vi "Console Example.vi"() -> ()   [LabVIEW 2020, in "ase.console.lvlib"]
uses:
  ase.console.lvlib
  <vilib>/Utility/miscctls.llb/LVPointTypeDef.ctl
  ase/ase/ase.lvclass/ase.ctl
  ase/ase/Merge Call Library Errors.vi
  ase/ase/Trim Whitespace.vi
  ase/ase/Check Shared Library Version.vi
  ase/ase/Write Data to Std In.vi
  ase/ase/Error Invalid ASE Handle.vi
  ase/ase/Error Internal Library Implementation Error.vi
  <vilib>/Utility/error.llb/Error Cluster From Error Code.vi
  ase/ase/Wait on Call.vi
  ase/ase/ase.lvclass
panel:
  in  "Write Exit":bool
  in  "Clear Std Out":bool
  in  "Start Console":bool
  in  "Send Terminate":bool
  in  "Clear Std Err":bool
  in  "working directory":path=path "c:/"
  in  "Send":bool
  in  "Cmd":string="echo hello!" caption="Cmd In (can include multiple lines)"
  out "Std Err":string
  out "Std Out":string
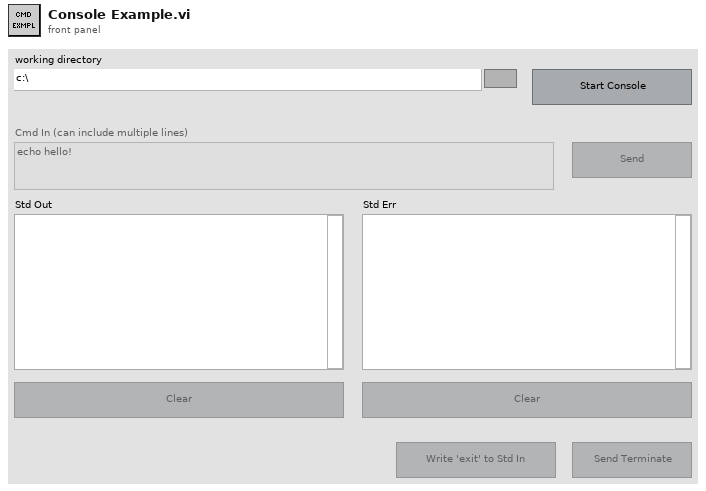
[diagram p1: front panel]
types:
  T1 = enum8{"Enabled", "Disabled", "Disabled and Grayed Out"}
  T2 = typedef "LVPointTypeDef.ctl" = cluster{"Horizontal":i16, "Vertical":i16}
  T3 = typedef "ase.lvlib/ase.lvclass/Event References.ctl" = cluster{"Standard Output":refnum<user-event>, "Standard Error":refnum<user-event>, "Did Exit":refnum<user-event>}
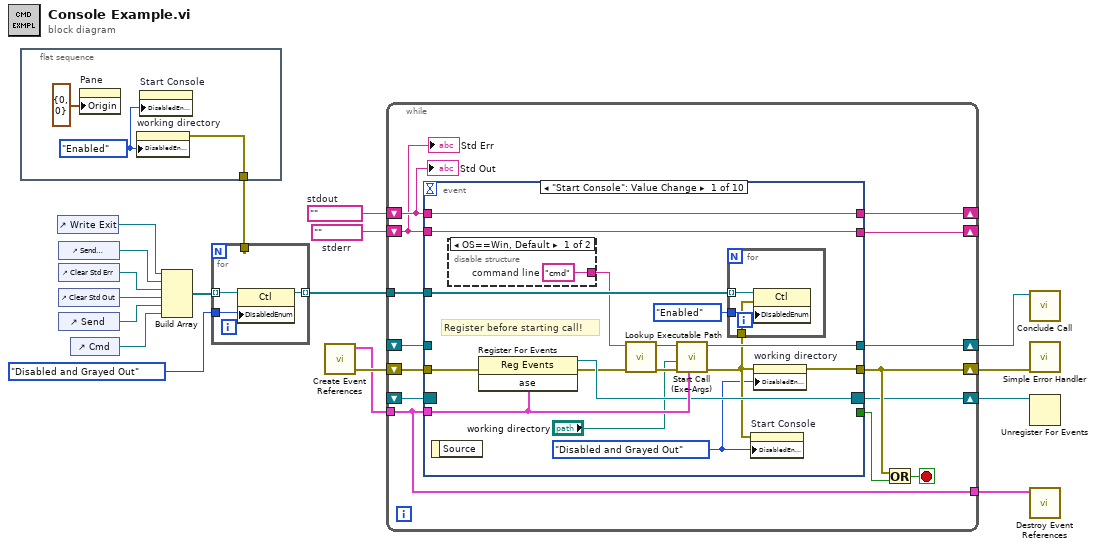
[diagram p0: block diagram]
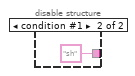
[diagram p2: hidden frame]
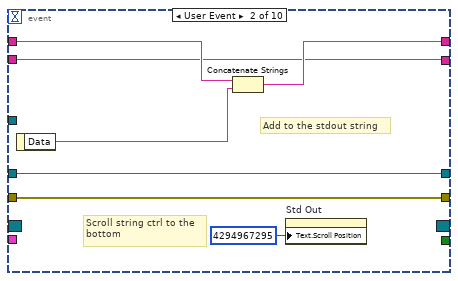
[diagram p3: hidden frame]
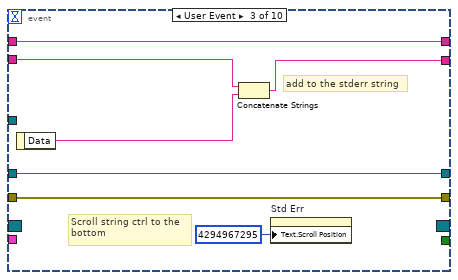
[diagram p4: hidden frame]
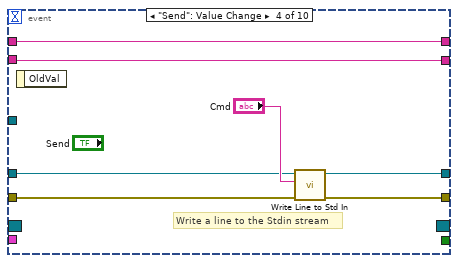
[diagram p5: hidden frame]
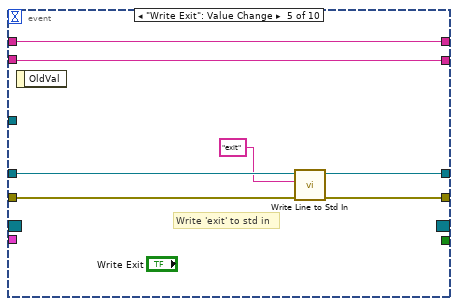
[diagram p6: hidden frame]
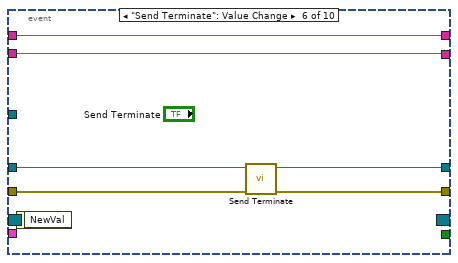
[diagram p7: hidden frame]
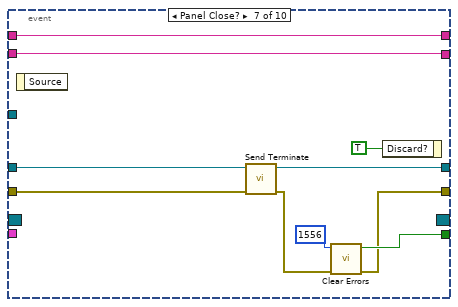
[diagram p8: hidden frame]
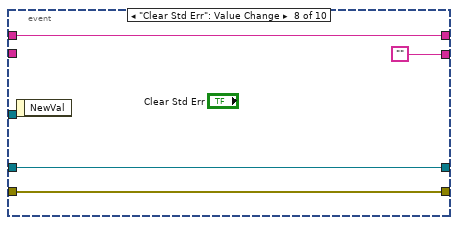
[diagram p9: hidden frame]
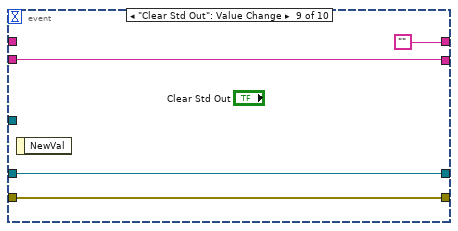
[diagram p10: hidden frame]
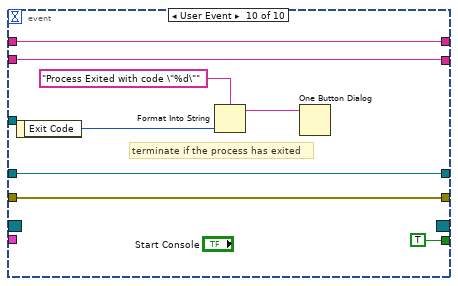
[diagram p11: hidden frame]
diagram:
  w12 = ""  # stderr
  w13 = ""  # stdout
  n1 = flat-sequence {
    tunnel: [w21] -> w3
    frame #0 {
      w19 = T1."Enabled" ("Disabled")
      n2 = property on="Pane" class="Pane"("Origin"=T2 {"Horizontal"=0, "Vertical"=0}) -> ()  [unwired: 2 in, 2 out]
      n3 = property on="working directory" class="Path"("DisabledEnum"=w19) -> (error out=w21:errorcluster)  [unwired: 2 in, 1 out]
      n4 = property on="Start Console" class="Bool"("DisabledEnum"=w19) -> ()  [unwired: 2 in, 2 out]
    }
  }
  n5 = control-ref of="Write Exit"() -> (w2:refnum<vi>)
  n6 = control-ref of="Send Terminate"() -> (w11:refnum<vi>)
  n7 = control-ref of="Clear Std Err"() -> (w10:refnum<vi>)
  n8 = control-ref of="Clear Std Out"() -> (w9:refnum<vi>)
  n9 = control-ref of="Send"() -> (w8:refnum<vi>)
  n10 = control-ref of="Cmd"() -> (w7:refnum<vi>)
  n11 = Build Array(w2, w11, w10, w9, w8, w7) -> (w6:refnum<vi>[])
  n12 = for {
    tunnel: w6 -> [w24] mode=indexing
    tunnel: T1."Disabled and Grayed Out" ("Disabled") -> [w23]
    tunnel: [w22] -> w4 mode=indexing
    tunnel: w3 -> [_]
    n13 = property class="Ctl"(reference=w24, "DisabledEnum"=w23) -> (reference out=w22:refnum<vi>)  [unwired: 1 in, 1 out]
  }
  n14 = call "Create Event References.vi"() -> ("error out"=w18:errorcluster, "ase"=w15:T3)  [unwired: 10 in]
  n15 = while {
    shift-right: [w36] -> w16
    shift-left: _ -> [w35]
    shift-right: [w37] -> w1
    shift-left: w18 -> [w38]
    shift-right: [w33] -> _
    shift-left: w13 -> [w27]
    shift-right: [w30] -> _
    shift-left: w12 -> [w26]
    tunnel: w15 -> [w29]
    tunnel: [w29] -> w14
    shift-right: [w34] -> w17
    shift-left: _ -> [w28]
    tunnel: w4 -> [w25]
    stop <- w31 stop-if-true
    n16 = event shown="[0] \"Start Console\": Value Change" {
      selector: w28 -> [_ _ _ _ _ _ _ _ _ _]
      dyn-events: [w48 _ _ _ _ _ _ _ _ _] -> w34
      timeout: _ -> [_ _ _ _ _ _ _ _ _ _]
      tunnel: [w51 w65 w72 w78 w85 w88 w100 w106 w111 w116] -> w36
      tunnel: w35 -> [_ w65 w72 w74 w82 w89 w101 w106 w111 w116]
      tunnel: w38 -> [w50 w66 w73 w79 w86 w93 w97 w107 w110 w119]
      tunnel: [w45 w66 w73 w80 w87 w92 w94 w107 w110 w119] -> w37
      tunnel: w27 -> [w53 w63 w69 w76 w84 w91 w103 w105 _ w117]
      tunnel: [w53 w64 w69 w76 w84 w91 w103 w105 "" w117] -> w33
      tunnel: [_ _ _ _ _ _ w95 _ _ TRUE] -> w32
      tunnel: w26 -> [w52 w61 w70 w75 w83 w90 w102 _ w109 w118]
      tunnel: [w52 w61 w68 w75 w83 w90 w102 "" w109 w118] -> w30
      tunnel: w29 -> [w49 _ _ _ _ _ _ _ _ _]
      tunnel: w25 -> [w46 _ _ _ _ _ _ _ _ _]
      event "Start Console": Value Change {
        w43 = T1."Disabled and Grayed Out" ("Disabled")
        # "Register before starting call!"
        n17 = event-data() -> ()  [unwired: 1 in, 1 out]
        n18 = disable-structure "Conditional Disable Structure" shown="OS==Win, Default" {
          disable-tunnel: [w58 "sh" ("command line")] -> w42
          frame condition #0 (active) {
            w58 = "cmd"  # command line
          }
          frame condition #1 {
          }
        }
        n19 = register-events(error in=w50, w49) -> (reference out=w48:refnum<event-registration>, error out=w41:errorcluster)  [unwired: 1 in]
        n20 = call "Lookup Executable Path.vi"("error in"=w41, "Executable Name"=w42) -> ("error out"=w54:errorcluster, "Path"=w40:path)  [unwired: 7 in, 1 out]
        n21 = call "Start Call (Exe-Args).vi"("Event References"=w49, "error in"=w54, "Working Directory (default <Not A Path> - System Default)"="working directory", "Executable Path"=w40) -> ("error out"=w44:errorcluster, "New ASE Handle"=w51:refnum<class "ase.lvclass">)  [unwired: 6 in]
        n22 = for {
          tunnel: w46 -> [w57] mode=indexing
          tunnel: T1."Enabled" ("Disabled") -> [w56]
          tunnel: w44 -> [w55]
          n23 = property class="Ctl"(reference=w57, error in=w55, "DisabledEnum"=w56) -> ()  [unwired: 2 out]
        }
        n24 = property on="Start Console" class="Bool"(error in=w44, "DisabledEnum"=w43) -> ()  [unwired: 1 in, 2 out]
        n25 = property on="working directory" class="Path"(error in=w44, "DisabledEnum"=w43) -> (error out=w45:errorcluster)  [unwired: 1 in, 1 out]
      }
      event User Event {
        # "Scroll string ctrl to the \nbottom"
        # "Add to the stdout string"
        n26 = event-data() -> ("Data"=w62:string)  [unwired: 1 in]
        n27 = Concatenate Strings(w63, w62) -> (w64:string)
        n28 = property on="Std Out" class="Str"("Text.Scroll Position"=u32 4294967295) -> ()  [unwired: 2 in, 2 out]
      }
      event User Event {
        # "Scroll string ctrl to the \nbottom"
        # "add to the stderr string"
        n29 = event-data() -> ("Data"=w71:string)  [unwired: 1 in]
        n30 = Concatenate Strings(w70, w71) -> (w68:string)
        n31 = property on="Std Err" class="Str"("Text.Scroll Position"=u32 4294967295) -> ()  [unwired: 2 in, 2 out]
      }
      event "Send": Value Change {
        # "Write a line to the Stdin stream"
        n32 = event-data() -> ()  [unwired: 1 in, 1 out]
        n33 = call "Write Line to Std In .vi"("error in"=w79, "Input"="Cmd", "ASE Handle"=w74) -> ("error out"=w80:errorcluster, "ASE Handle Duplicate"=w78:refnum<class "ase.lvclass">)  [unwired: 6 in, 1 out]
      }
      event "Write Exit": Value Change {
        # "Write 'exit' to std in"
        n34 = event-data() -> ()  [unwired: 1 in, 1 out]
        n35 = call "Write Line to Std In .vi"("error in"=w86, "Input"="exit", "ASE Handle"=w82) -> ("error out"=w87:errorcluster, "ASE Handle Duplicate"=w85:refnum<class "ase.lvclass">)  [unwired: 6 in, 1 out]
      }
      event "Send Terminate": Value Change {
        n36 = event-data() -> ()  [unwired: 1 in, 1 out]
        n37 = call "Send Terminate.vi"("error in"=w93, "ASE Handle"=w89) -> ("error out"=w92:errorcluster, "ASE Handle Duplicate"=w88:refnum<class "ase.lvclass">)  [unwired: 7 in, 1 out]
      }
      event Panel Close? {
        n38 = event-data() -> ()  [unwired: 1 in, 1 out]
        n39 = call "Send Terminate.vi"("error in"=w97, "ASE Handle"=w101) -> ("error out"=w98:errorcluster, "ASE Handle Duplicate"=w100:refnum<class "ase.lvclass">)  [unwired: 7 in, 1 out]
        n40 = call <vilib>:"Clear Errors.vi"("error in (no error)"=w98, "specific error code to clear (0: all)"=1556) -> ("error out"=w94:errorcluster, "specific error cleared?"=w95:bool)  [unwired: 4 in]
        n41 = event-data("Discard?"=TRUE) -> ()  [unwired: 1 in, 1 out]
      }
      event "Clear Std Err": Value Change {
        n42 = event-data() -> ()  [unwired: 1 in, 1 out]
      }
      event "Clear Std Out": Value Change {
        n43 = event-data() -> ()  [unwired: 1 in, 1 out]
      }
      event User Event {
        # "terminate if the process has exited"
        n44 = event-data() -> ("Exit Code"=w114:i32)  [unwired: 1 in]
        n45 = Format Into String(format string="Process Exited with code \"%d\"", w114) -> (resulting string=w113:string)  [unwired: 2 in, 1 out]
        n46 = One Button Dialog(message=w113) -> ()  [unwired: 1 in, 1 out]
      }
    }
    n47 = Or(x=w37, y=w32) -> (x .or. y?=w31:bool)
    "Std Err" <- w26
    "Std Out" <- w27
  }
  n48 = call "Conclude Call.vi"("ASE Handle"=w16) -> ()  [unwired: 8 in, 3 out]
  n49 = call <vilib>:"Simple Error Handler.vi"("error in (no error)"=w1) -> ()  [unwired: 4 in, 5 out]
  n50 = Unregister For Events(event registration refnum=w17) -> ()  [unwired: 1 in, 1 out]
  n51 = call "Destroy Event References.vi"("Event References"=w14) -> ()  [unwired: 10 in, 1 out]
